vi "Compute Shared Key.vi"(9 "GUID":string, 10 "SecretKey":string) -> (2 "Shared Key":string)   [LabVIEW 2013, in "Attribute.Owner.lvclass"]
uses:
  Attribute.Owner.lvclass
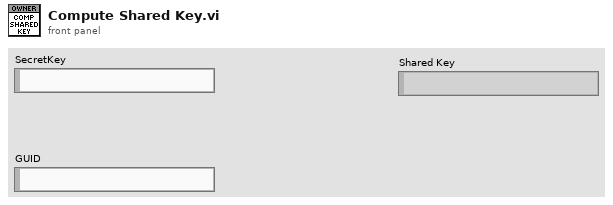
[diagram p1: front panel]
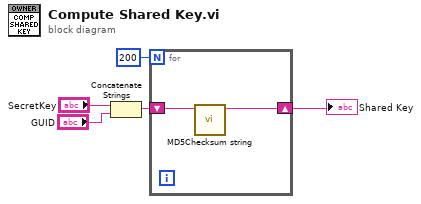
[diagram p0: block diagram]
diagram:
  n1 = Concatenate Strings("SecretKey", "GUID") -> (w3:string)
  n2 = for {
    N: 200 -> [_]
    shift-right: [w6] -> w2
    shift-left: w3 -> [w7]
    n3 = call <vilib>:"MD5Checksum string.vi"("Message String"=w7) -> ("MD5 message-digest"=w6:string)  [unwired: 10 in]
  }
  "Shared Key" <- w2
